vi "WriteAuxLockin.vi"(0 "Output #":i32=1, 1 "Voltage":dbl=1.0 step=0.01, 2 "VISA resource name":refnum<visa-resource-name>="COM5") -> ()   [LabVIEW 2013]
uses:
  <vilib>/Instr/_visa.llb/VISA Configure Serial Port (Instr).vi
panel:
  in  "flow control":u16(ring) items=["None"=0, "XON/XOFF"=1, "RTS/CTS"=2, "DTR/DSR"=4]
  in  "stop bits":u16(ring)=10 items=["1.0"=10, "1.5"=15, "2.0"=20]
  in  "parity":u16(ring) items=["None", "Odd", "Even", "Mark", "Space"]
  in  "data bits":u16=8 min=5 max=8 step=1
  in  "baud rate":u32=9600
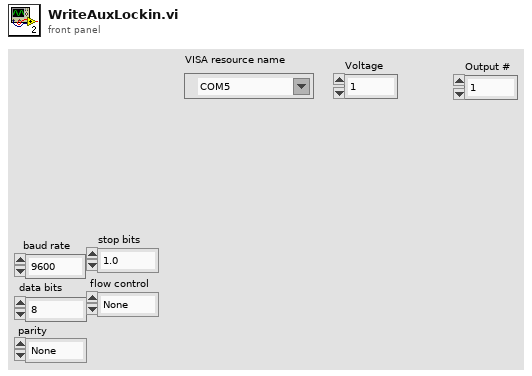
[diagram p1: front panel]
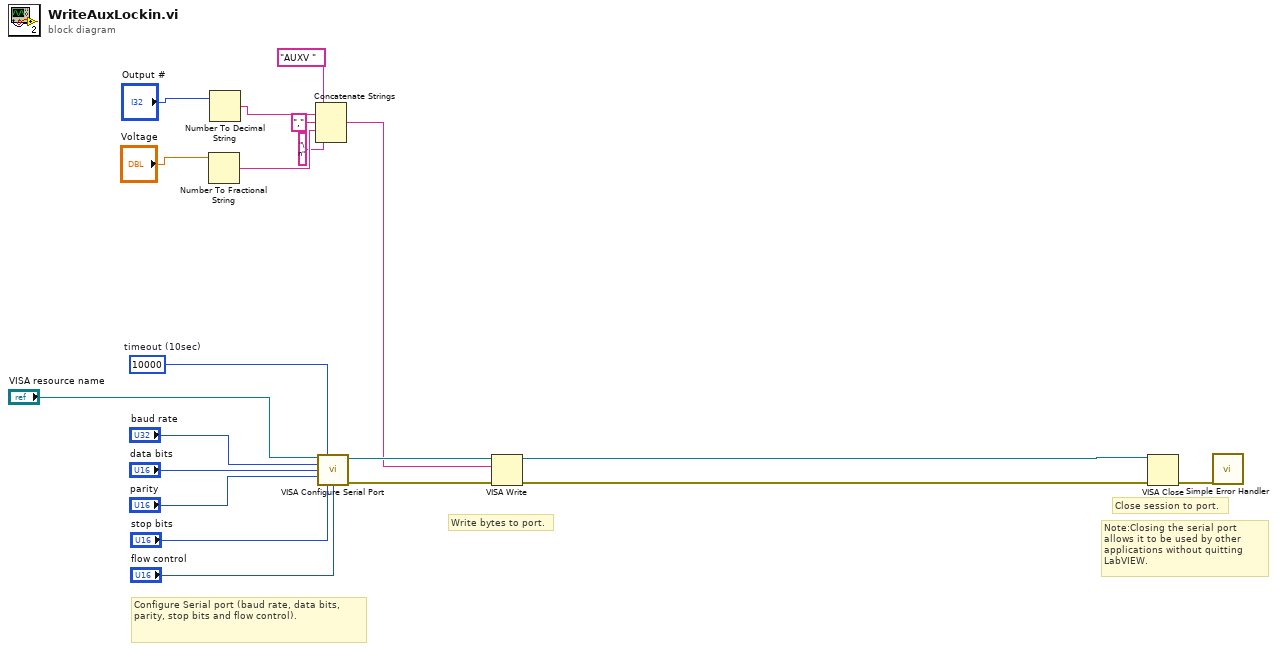
[diagram p0: block diagram]
diagram:
  w14 = u32 10000  # timeout (10sec)
  # "Write bytes to port."
  # "Note:Closing the serial port allows it to be used by other applications without quitting LabVIEW."
  # "Configure Serial port (baud rate, data bits, parity, stop bits and flow control)."
  # "Close session to port."
  n1 = Number To Fractional String(number="Voltage") -> (F-format string=w5:string)  [unwired: 3 in]
  n2 = Number To Decimal String(number="Output #") -> (decimal integer string=w7:string)  [unwired: 1 in]
  n3 = Concatenate Strings("AUXV ", w7, "," ("string"), w5, "\n" ("string")) -> (w3:string)
  n4 = call-poly "VISA Configure Serial Port"("VISA resource name"="VISA resource name", "timeout (10sec)"=w14, "baud rate (9600)"="baud rate", "data bits (8)"="data bits", "parity (0:none)"="parity", "stop bits (10: 1 bit)"="stop bits", "flow control (0:none)"="flow control") -> ("VISA resource name out"=w17:refnum<visa-resource-name>, "error out"=w18:errorcluster)  [unwired: 2 in, 5 out]
  n5 = VISA Write(VISA resource name=w17, write buffer=w3, error in (no error)=w18) -> (VISA resource name out=w2:refnum<visa-resource-name>, error out=w1:errorcluster)  [unwired: 1 out]
  n6 = VISA Close(VISA resource name=w2, error in (no error)=w1) -> (error out=w16:errorcluster)
  n7 = call <vilib>:"Simple Error Handler.vi"("error in (no error)"=w16) -> ()  [unwired: 1 in, 8 out]
